vi "st_Hypergeometric PDF (kx).vi"(8 "n = samples drawn":i32=20, 9 "k = items":i32=30, 10 "M = size of population":i32=100, 11 "x":dbl=1.0) -> (0 "error":i32, 3 "pdf(x)":dbl=0.003553328058550957)   [LabVIEW 2018, in "NI_Gmath.lvlib"]
uses:
  NI_Gmath.lvlib
  st_error_code.ctl
panel:
  # "Hypergeometric PDF (kx)"
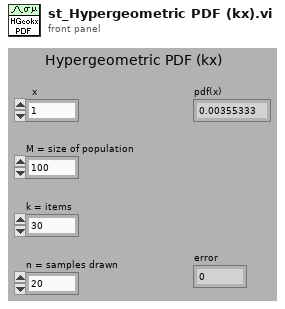
[diagram p1: front panel]
types:
  T1 = typedef "NI_Gmath.lvlib/st_error_code.ctl" = i32
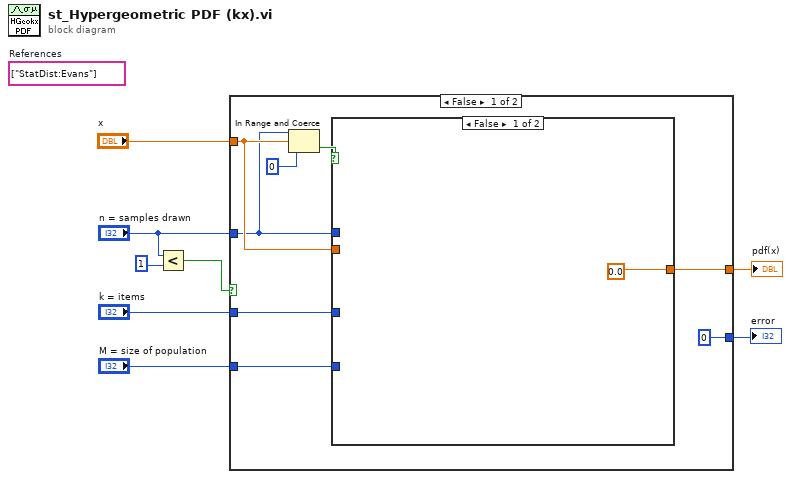
[diagram p0: block diagram]
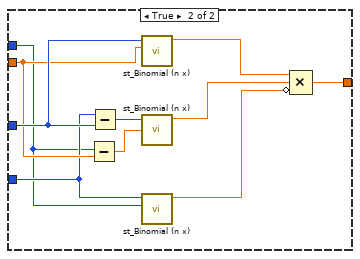
[diagram p2: hidden frame]
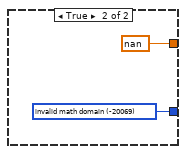
[diagram p3: hidden frame]
diagram:
  (unwired) string[] ["StatDist:Evans"]  # References
  n1 = Less?(x="n = samples drawn", y=1) -> (x < y?=w4:bool)
  n2 = case shown="False" w4 {
    tunnel: [0 ("invalid math domain") w28] -> w8
    tunnel: [w12 nan] -> w7
    tunnel: "x" -> [w14 _]
    tunnel: "n = samples drawn" -> [w13 _]
    tunnel: "k = items" -> [w10 _]
    tunnel: "M = size of population" -> [w9 _]
    frame False {
      n3 = In Range and Coerce(upper limit=w13, x=w14, lower limit=0) -> (In Range?=w11:bool)  [unwired: 1 out]
      n4 = case shown="False" w11 {
        tunnel: [0.0 w18] -> w12
        tunnel: w14 -> [_ w25]
        tunnel: w13 -> [_ w21]
        tunnel: w10 -> [_ w26]
        tunnel: w9 -> [_ w22]
        frame False {
        }
        frame True {
          n5 = Subtract(x=w21, y=w25) -> (x-y=w23:dbl)
          n6 = Subtract(x=w22, y=w26) -> (x-y=w24:i32)
          n7 = call "st_Binomial (n x).vi"("x"=w25, "n"=w26) -> ("binomial (n x)"=w27:dbl)  [unwired: 8 in, 1 out]
          n8 = call "st_Binomial (n x).vi"("x"=w23, "n"=w24) -> ("binomial (n x)"=w20:dbl)  [unwired: 8 in, 1 out]
          n9 = call "st_Binomial (n x).vi"("x"=w21, "n"=w22) -> ("binomial (n x)"=w19:dbl)  [unwired: 8 in, 1 out]
          n10 = Compound Arithmetic op=MULTIPLY(w27, w20, invert w19) -> (w18:dbl)
        }
      }
    }
    frame True {
      w28 = T1 -20069 items=["invalid math domain"=-20069, "Fourier interpolation size m >= n"=-20070, "empty array"=-20003] ("stat interp error code")
    }
  }
  "pdf(x)" <- w7
  "error" <- w8
